vi "Save data file to network drive v3.vi"(8 "Input Cluster":T1, 11 "panel id":string) -> (0 "network file save error":errorcluster, 3 "file save path":string)   [LabVIEW 2013]
uses:
  program files/Global 1.vi
panel:
  out "status":string
  out "C drive root path":string
  out "network file dir path":path
  out "network dir":string
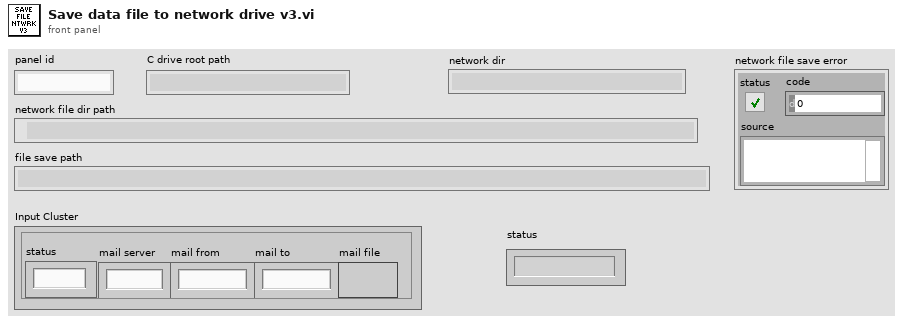
[diagram p1: front panel]
types:
  T1 = cluster{"status":string, "mail server":string, "mail from":string, "mail to":string, "mail file":bool}
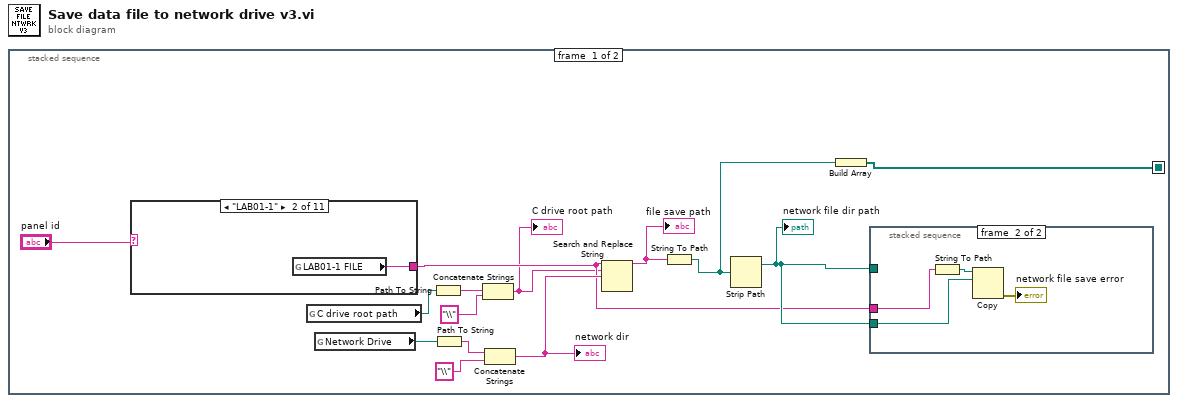
[diagram p0: block diagram]
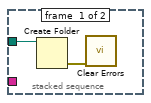
[diagram p2: hidden frame]
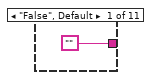
[diagram p3: hidden frame]
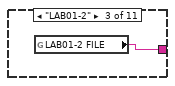
[diagram p4: hidden frame]
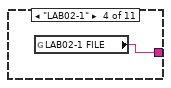
[diagram p5: hidden frame]
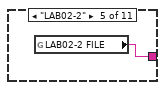
[diagram p6: hidden frame]
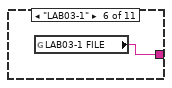
[diagram p7: hidden frame]
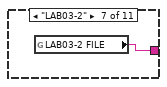
[diagram p8: hidden frame]
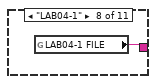
[diagram p9: hidden frame]
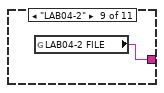
[diagram p10: hidden frame]
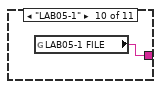
[diagram p11: hidden frame]
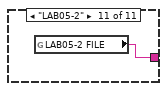
[diagram p12: hidden frame]
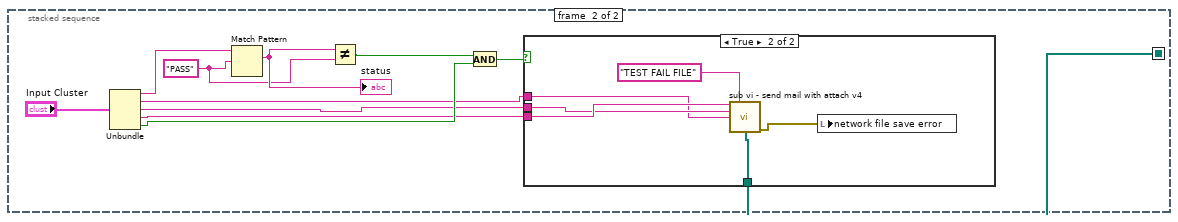
[diagram p13: hidden frame]
diagram:
  n1 = stacked-sequence {
    seq-local: [w1 _] -> [_ w32]
    frame #0 {
      n2 = case shown="\"LAB01-1\"" "panel id" {
        tunnel: ["" w22 w23 w24 w25 w26 w27 w28 w29 w30 w31] -> w7
        frame "False", Default {
        }
        frame "LAB01-1" {
          n3 = global read "Global 1.vi" "LAB01-1 FILE"() -> (w22:string)
        }
        frame "LAB01-2" {
          n4 = global read "Global 1.vi" "LAB01-2 FILE"() -> (w23:string)
        }
        frame "LAB02-1" {
          n5 = global read "Global 1.vi" "LAB02-1 FILE"() -> (w24:string)
        }
        frame "LAB02-2" {
          n6 = global read "Global 1.vi" "LAB02-2 FILE"() -> (w25:string)
        }
        frame "LAB03-1" {
          n7 = global read "Global 1.vi" "LAB03-1 FILE"() -> (w26:string)
        }
        frame "LAB03-2" {
          n8 = global read "Global 1.vi" "LAB03-2 FILE"() -> (w27:string)
        }
        frame "LAB04-1" {
          n9 = global read "Global 1.vi" "LAB04-1 FILE"() -> (w28:string)
        }
        frame "LAB04-2" {
          n10 = global read "Global 1.vi" "LAB04-2 FILE"() -> (w29:string)
        }
        frame "LAB05-1" {
          n11 = global read "Global 1.vi" "LAB05-1 FILE"() -> (w30:string)
        }
        frame "LAB05-2" {
          n12 = global read "Global 1.vi" "LAB05-2 FILE"() -> (w31:string)
        }
      }
      n13 = global read "Global 1.vi" "C drive root path"() -> (w4:path)
      n14 = global read "Global 1.vi" "Network Drive"() -> (w13:path)
      n15 = Path To String(path=w4) -> (string=w5:string)
      n16 = Path To String(path=w13) -> (string=w12:string)
      n17 = Concatenate Strings(w5, "\\") -> (w3:string)
      "C drive root path" <- w3
      n18 = Concatenate Strings(w12, "\\") -> (w10:string)
      "network dir" <- w10
      n19 = Search and Replace String(input string=w7, search string=w3, replace string=w10) -> (result string=w9:string)  [unwired: 5 in, 3 out]
      "file save path" <- w9
      n20 = String To Path(string=w9) -> (path=w2:path)
      n21 = Strip Path(path=w2) -> (stripped path=w8:path)  [unwired: 1 out]
      "network file dir path" <- w8
      n22 = Build Array(w2) -> (w1:path[])
      n23 = stacked-sequence {
        tunnel: w8 -> [w16 _]
        tunnel: w7 -> [_ w18]
        tunnel: w8 -> [_ w17]
        frame #0 {
          n24 = Create Folder(path (use dialog)=w16) -> (error out=w15:errorcluster)  [unwired: 2 in, 2 out]
          n25 = call <vilib>:"Clear Errors.vi"("error in (no error)"=w15) -> ()  [unwired: 6 in, 1 out]
        }
        frame #1 {
          n26 = String To Path(string=w18) -> (path=w19:path)
          n27 = Copy(10:w17, 11:w19) -> (0:→"network file save error":errorcluster)  [unwired: 3 in, 2 out]
        }
      }
    }
    frame #1 {
      w37 = "PASS"
      n28 = Unbundle("Input Cluster") -> ("status"=w39:string, "mail server"=w33:string, "mail from"=w34:string, "mail to"=w35:string, "mail file"=w40:bool)
      n29 = Match Pattern(string=w39, regular expression=w37) -> (match substring=w38:string)  [unwired: 1 in, 3 out]
      "status" <- w38
      n30 = Not Equal?(x=w38, y=w37) -> (x != y?=w36:bool)
      n31 = And(x=w36, y=w40) -> (x .and. y?=w42:bool)
      n32 = case shown="True" w42 {
        tunnel: w35 -> [_ w47]
        tunnel: w34 -> [_ w46]
        tunnel: w33 -> [_ w45]
        tunnel: w32 -> [_ w44]
        frame False {
        }
        frame True {
          n33 = call "sub vi - send mail with attach v4.vi"("TO:"=w47, "subject"="TEST FAIL FILE", "from"=w46, "out going server"=w45, "Attachements"=w44) -> ("error out"=w48:errorcluster)  [unwired: 10 in]
          n34 = local write "network file save error"(w48) -> ()
        }
      }
    }
  }
